vi "About Box.vi"(1 "error in (no error)":errorcluster) -> (0 "error out":errorcluster)   [LabVIEW 2018]
uses:
  Type Defs/RT Command.ctl
  FGVs/Global Variables.vi
panel:
  in  "OK":bool
  out "Software version":string="Ionica Firmware; FPGA: 277101103; RT: 341101125\n(System is idling: 0h3m24s)"
  out "version":string="Ionica Firmware; FPGA: 277101103; RT: 341101125\n(System is idling: 0h3m24s)"
  # "Copyright ©Aug 2020\nPerkin Elmer Canada\nAll Right Reserved\n\nAll Right Reserved"
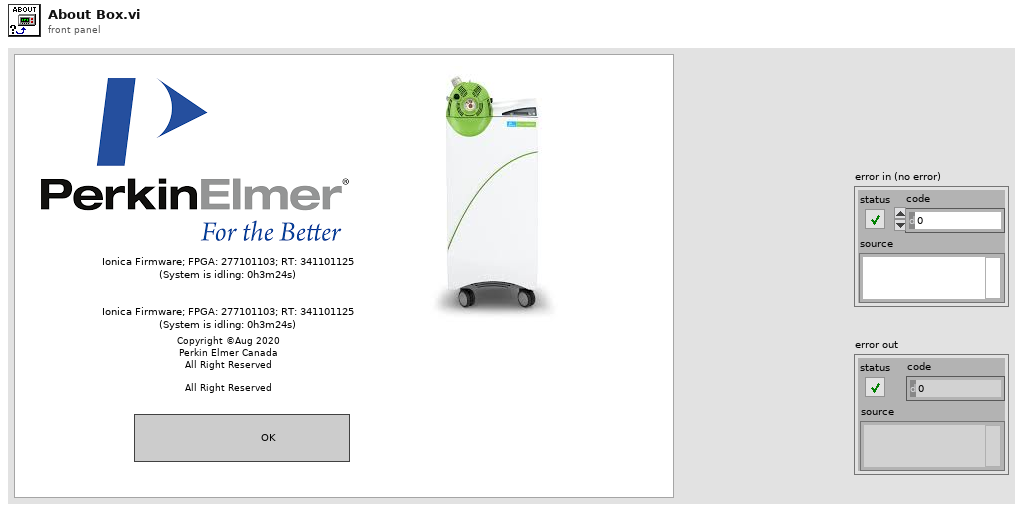
[diagram p1: front panel]
types:
  T1 = typedef "RT Command.ctl" = enum16{"xml Start Run", "xml Start Actual Run", "xml Stop Run", "xml Runtime Update", "xml Get Status", "xml Get Table", "xml Set Table", "xml Get Configuration", "xml System Status", "xml Set LC Input Logic", "xml Get Data", "xml Get Info", "Start", "StartActualRun", "Stop", "Runtime Update", "Get Data", "Get Info", "Get Status", "Get Param", "Get Config", "Get Table", "Read ADC", "Set Oscillator", "Update Config", "Update Table", "Set All Pol", "Set Pol and DC", "Set Max Mass", "Toggle RP", "Toggle EL", "Set PIC", "Initialize Turbo", "Send Turbo Comm", "Close Turbo", "P1", "P2", "P3", "Send Serial", "Set LC Out", "Get LC In", "Read VAC", "Test Table", "Toggle Power", "Get Startup", "Set Startup", "Get ADC Table", "Set ADC Table", "Get Brief Status", "Get Detail Status", "Auxiliary Update", "Set CC Logics", "Set CC Input Logics", "Ignore Error", "invalid"}
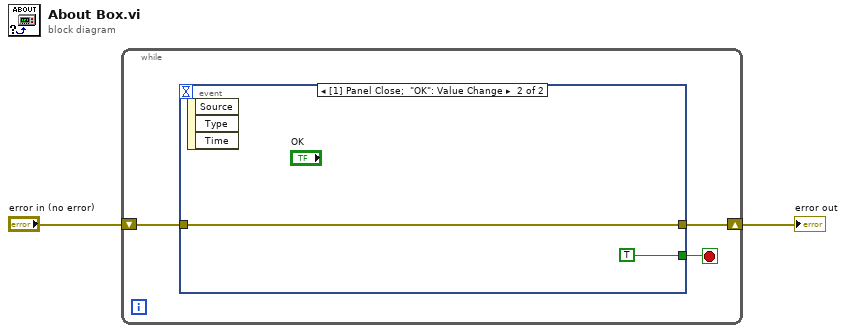
[diagram p0: block diagram]
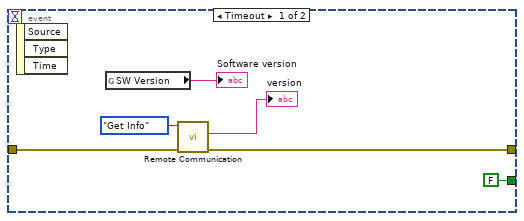
[diagram p2: hidden frame]
diagram:
  n1 = while {
    shift-right: [w4] -> w1
    shift-left: "error in (no error)" -> [w5]
    stop <- w3 stop-if-true
    n2 = event shown="[1] Panel Close;  \"OK\": Value Change" {
      selector: _ -> [_ _]
      dyn-events: _ -> [_ _]
      timeout: _ -> [_ _]
      tunnel: w5 -> [w11 w12]
      tunnel: [w10 w12] -> w4
      tunnel: [FALSE TRUE] -> w3
      event Timeout {
        n3 = event-data() -> ()  [unwired: 1 in, 3 out]
        n4 = global read "Global Variables.vi" "SW Version"() -> (→"Software version":string)
        n5 = call "Remote Communication.vi"("Error In"=w11, "Command"=RT_Command."Get Info") -> ("Error Out"=w10:errorcluster, "Info"=→"version":string)  [unwired: 4 in, 2 out]
      }
      event Panel Close; "OK": Value Change {
        n6 = event-data() -> ()  [unwired: 1 in, 3 out]
      }
    }
  }
  "error out" <- w1
